vi "Settings.vi"(8 "error in (no error)":errorcluster, 11 "Pick and Place.lvclass":refnum<class "Pick and Place.lvclass">) -> (0 "error out":errorcluster, 3 "Pick and Place.lvclass 2":refnum<class "Pick and Place.lvclass">)   [LabVIEW 2020, in "Pick and Place.lvclass"]
uses:
  Pick and Place.lvclass
  Pick and Place Type.ctl
  Pick and Place.lvclass/Pick and Place.ctl
panel:
  in  "Pick and Place Type":T1
  in  "OK Button":bool
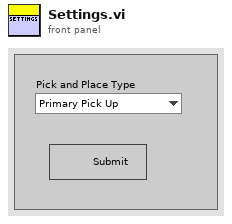
[diagram p1: front panel]
types:
  T1 = typedef "Pick and Place.lvclass/Pick and Place Type.ctl" = enum16{"Primary Pick Up", "Secondary Pick Up", "Put Down All", "Pick Up All", "Put Down Secondary"}
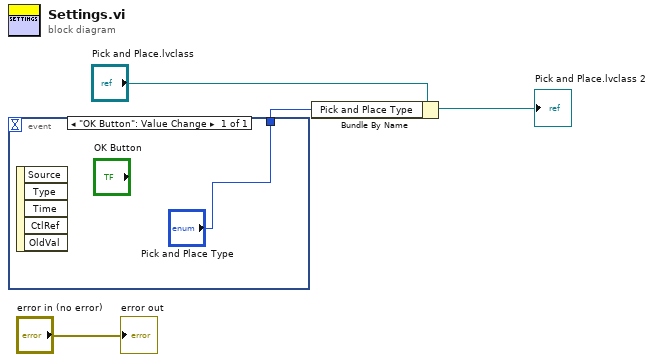
[diagram p0: block diagram]
diagram:
  n1 = event shown="[0] \"OK Button\": Value Change" {
    selector: _ -> [_]
    dyn-events: _ -> [_]
    timeout: _ -> [_]
    tunnel: ["Pick and Place Type"] -> w1
    event "OK Button": Value Change {
      n2 = event-data() -> ()  [unwired: 1 in, 5 out]
    }
  }
  n3 = Bundle By Name(cluster="Pick and Place.lvclass", "Pick and Place Type"=w1) -> (→"Pick and Place.lvclass 2":refnum<class "Pick and Place.lvclass">)
  "error out" <- "error in (no error)"
